vi "5G_PHY_PUSCH_main.vi"() -> ()   [LabVIEW 2015]
uses:
  <vilib>/Utility/miscctls.llb/LVBoundsTypeDef.ctl
  <vilib>/measure/maspectr.llb/FFT Spectrum (Mag-Phase) for 1 Chan (CDB).vi
  <vilib>/measure/NI_MAPro.lvlib
panel:
  out "总比特数 （信宿比特）":dbl
  out "误码率（信源比特和信宿比特比较）":dbl
  out "总比特数（解调制映射输出数据）":dbl
  out "误码率（调制映射输入数据和解调制映射输出数据比较）":dbl
  in  "第1径和第2径相偏(rad)":dbl[](array[numeric])=[0.0, 1.0] min=0.0 max=3.14
  in  "第1径和第2径幅度":dbl[](array[numeric])=[1.0, 0.5] min=0.0 max=1.0
  in  "第1径和第2径频偏(Hz)":dbl[](array[numeric])=[20.0, 140.0] min=0.0 max=180.0
  in  "第1径和第2径时间延迟采样点":dbl[](array[numeric])=[10.0, 140.0] min=0.0 max=200.0
  in  "多径使能":u16(ring) items=["不使能", "使能"]
  out "CRC校验结果":bool
  out "导频2信道估计值":dbl[][](graph)
  out "导频1信道估计值":dbl[][](graph)
  out "OFDM调制后数据（I路）":dbl[](graph)
  out "资源映射后数据（I路）":dbl[][](graph)
  out "产生导频后数据（I路）":dbl[][](graph)
  in  "CP多径时延采样点":i32=140 caption="dB" min=50 max=150
  in  "CP多径时延开关":u16(ring) items=["关", "开"]
  out "接收图片":picture
  out "发送图片":picture
  out "发送信号波形（I路）":dbl[](graph)
  in  "是否添加噪声":u16(ring) items=["关", "开"]
  in  "同步开关":u16(ring)=1 items=["关", "开"]
  in  "频偏(Hz)":i32=120 caption="dB" min=50 max=200
  in  "频偏开关":u16(ring) items=["关", "开"]
  out "相关峰(同步开关打开时显示)":dbl[](graph)
  in  "选择接收图片地址":path=path "C:/Users/DELL/Desktop/5Gphysicallayerlink/01 TeacherVersion/MatlabCode/rx_img.bmp"
  in  "选择发送图片地址":path=path "C:/Users/DELL/Desktop/5Gphysicallayerlink/01 TeacherVersion/MatlabCode/tx_img.bmp"
  out "误码数（调制映射输入数据和解调制映射输出数据比较）":i32
  out "误码数（信源比特和信宿比特比较）":i32
  in  "收发延迟采样点":i32=1400 caption="dB" min=0 max=7000
  in  "收发时延开关":u16(ring) items=["关", "开"]
  in  "突发干扰时域长度":i32=800 caption="dB" min=500 max=1000
  in  "突发干扰开关":u16(ring) items=["关", "开"]
  in  "信道估计开关":u16(ring)=1 items=["关", "开"]
  in  "CP开关":u16(ring)=1 items=["关", "开"]
  in  "交织开关":u16(ring)=1 items=["关", "开"]
  in  "LDPC开关":dbl(ring)=1.0 items=["关", "开"]
  in  "SNR":dbl=17.0 caption="dB" min=-10.0 max=50.0
  out "接收信号波形（I路）":dbl[](graph)
  in  "XSRP IP":string="192.168.1.166"
  in  "PC IP":string="192.168.1.180"
  in  "运行方式":enum16{"仿真运行", "真实系统"}(ring)
  in  "发送参数":T1={"发送通道"=enum."TxCh1", "发送频率"=2380000000.0, "发射衰减 "=40} {"发送频率" format="%#_6p"}
  in  "接收参数":T2={"接收通道"=enum."RxCh1", "接收频率"=2380000000.0, "接收增益 "=20} {"接收频率" format="%#_6p"}
  in  "调制参数":T3={"Nl"=1.0, "subframe_type"=1.0, "cp_type"=0.0, "cfi"=1.0, "UL_subframe_num"=2.0, "prb_num"=100.0, "调制类型"=3, "mimo_type"=1.0} {"调制类型" items=["QPSK"=1, "16QAM"=2, "64QAM"=3, "256QAM"=4]}
  in  "添加噪声":i16(ring) items=["添加噪声"=1, "不添加噪声"=0]
  out "crc_flag":dbl
  out "发送端星座图":cdb[](graph)
  out "接收信号频谱":cluster{"f0":dbl, "df":dbl, "magnitude":dbl[]}(graph)
  out "接收端星座图":cdb[](graph)
  # "基于XSRP软件无线电平台的LTE无线通信系统"
  # "基于XSRP软件无线电平台的5G NR 无线通信系统设计"
  # "实验参数设置"
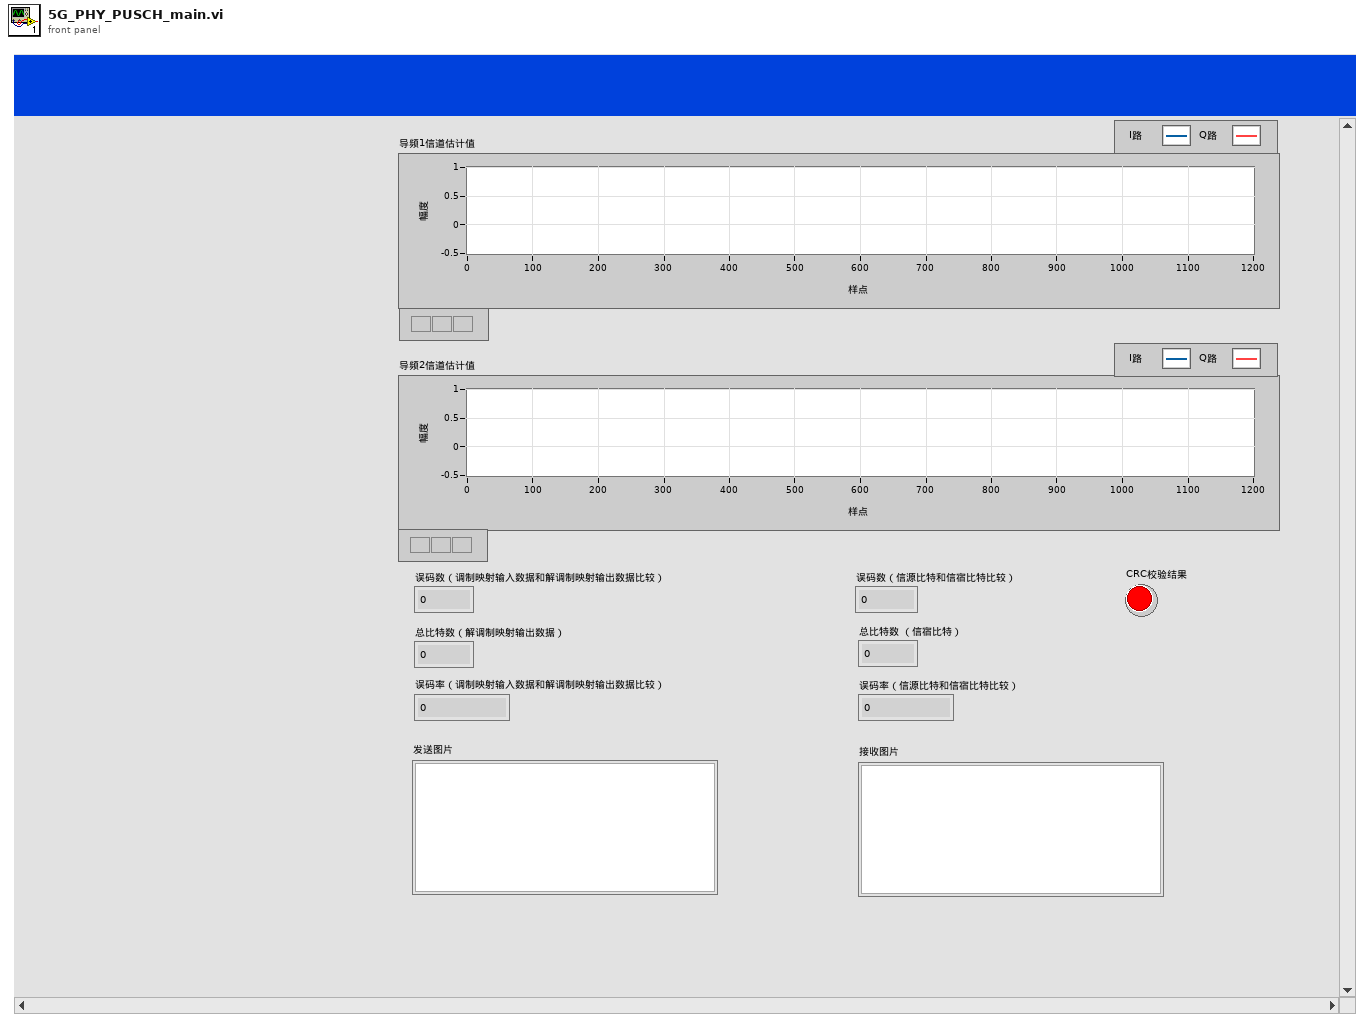
[diagram p1: front panel]
types:
  T1 = cluster{"发送通道":enum16{"TxCh1", "TxCh2"}, "发送频率":dbl, "发射衰减 ":u8}
  T2 = cluster{"接收通道":enum16{"RxCh1", "RxCh2"}, "接收频率":dbl, "接收增益 ":u8}
  T3 = cluster{"Nl":dbl, "subframe_type":dbl, "cp_type":dbl, "cfi":dbl, "UL_subframe_num":dbl, "prb_num":dbl, "调制类型":u16, "mimo_type":dbl}
  T4 = typedef "LVBoundsTypeDef.ctl" = cluster{"Width":u32, "Height":u32}
  T5 = cluster{"dB On (F)":bool, "unwrap phase (F)":bool, "convert to degree (F)":bool}
  T6 = enum8{"Enabled", "Disabled", "Disabled and Grayed Out"}
  T7 = typedef "imagedata.ctl" = cluster{"image type":i32, "image depth":i32, "image":u8[], "mask":u8[], "colors":u32[], "Rectangle":cluster{"left":i16, "top":i16, "right":i16, "bottom":i16}}
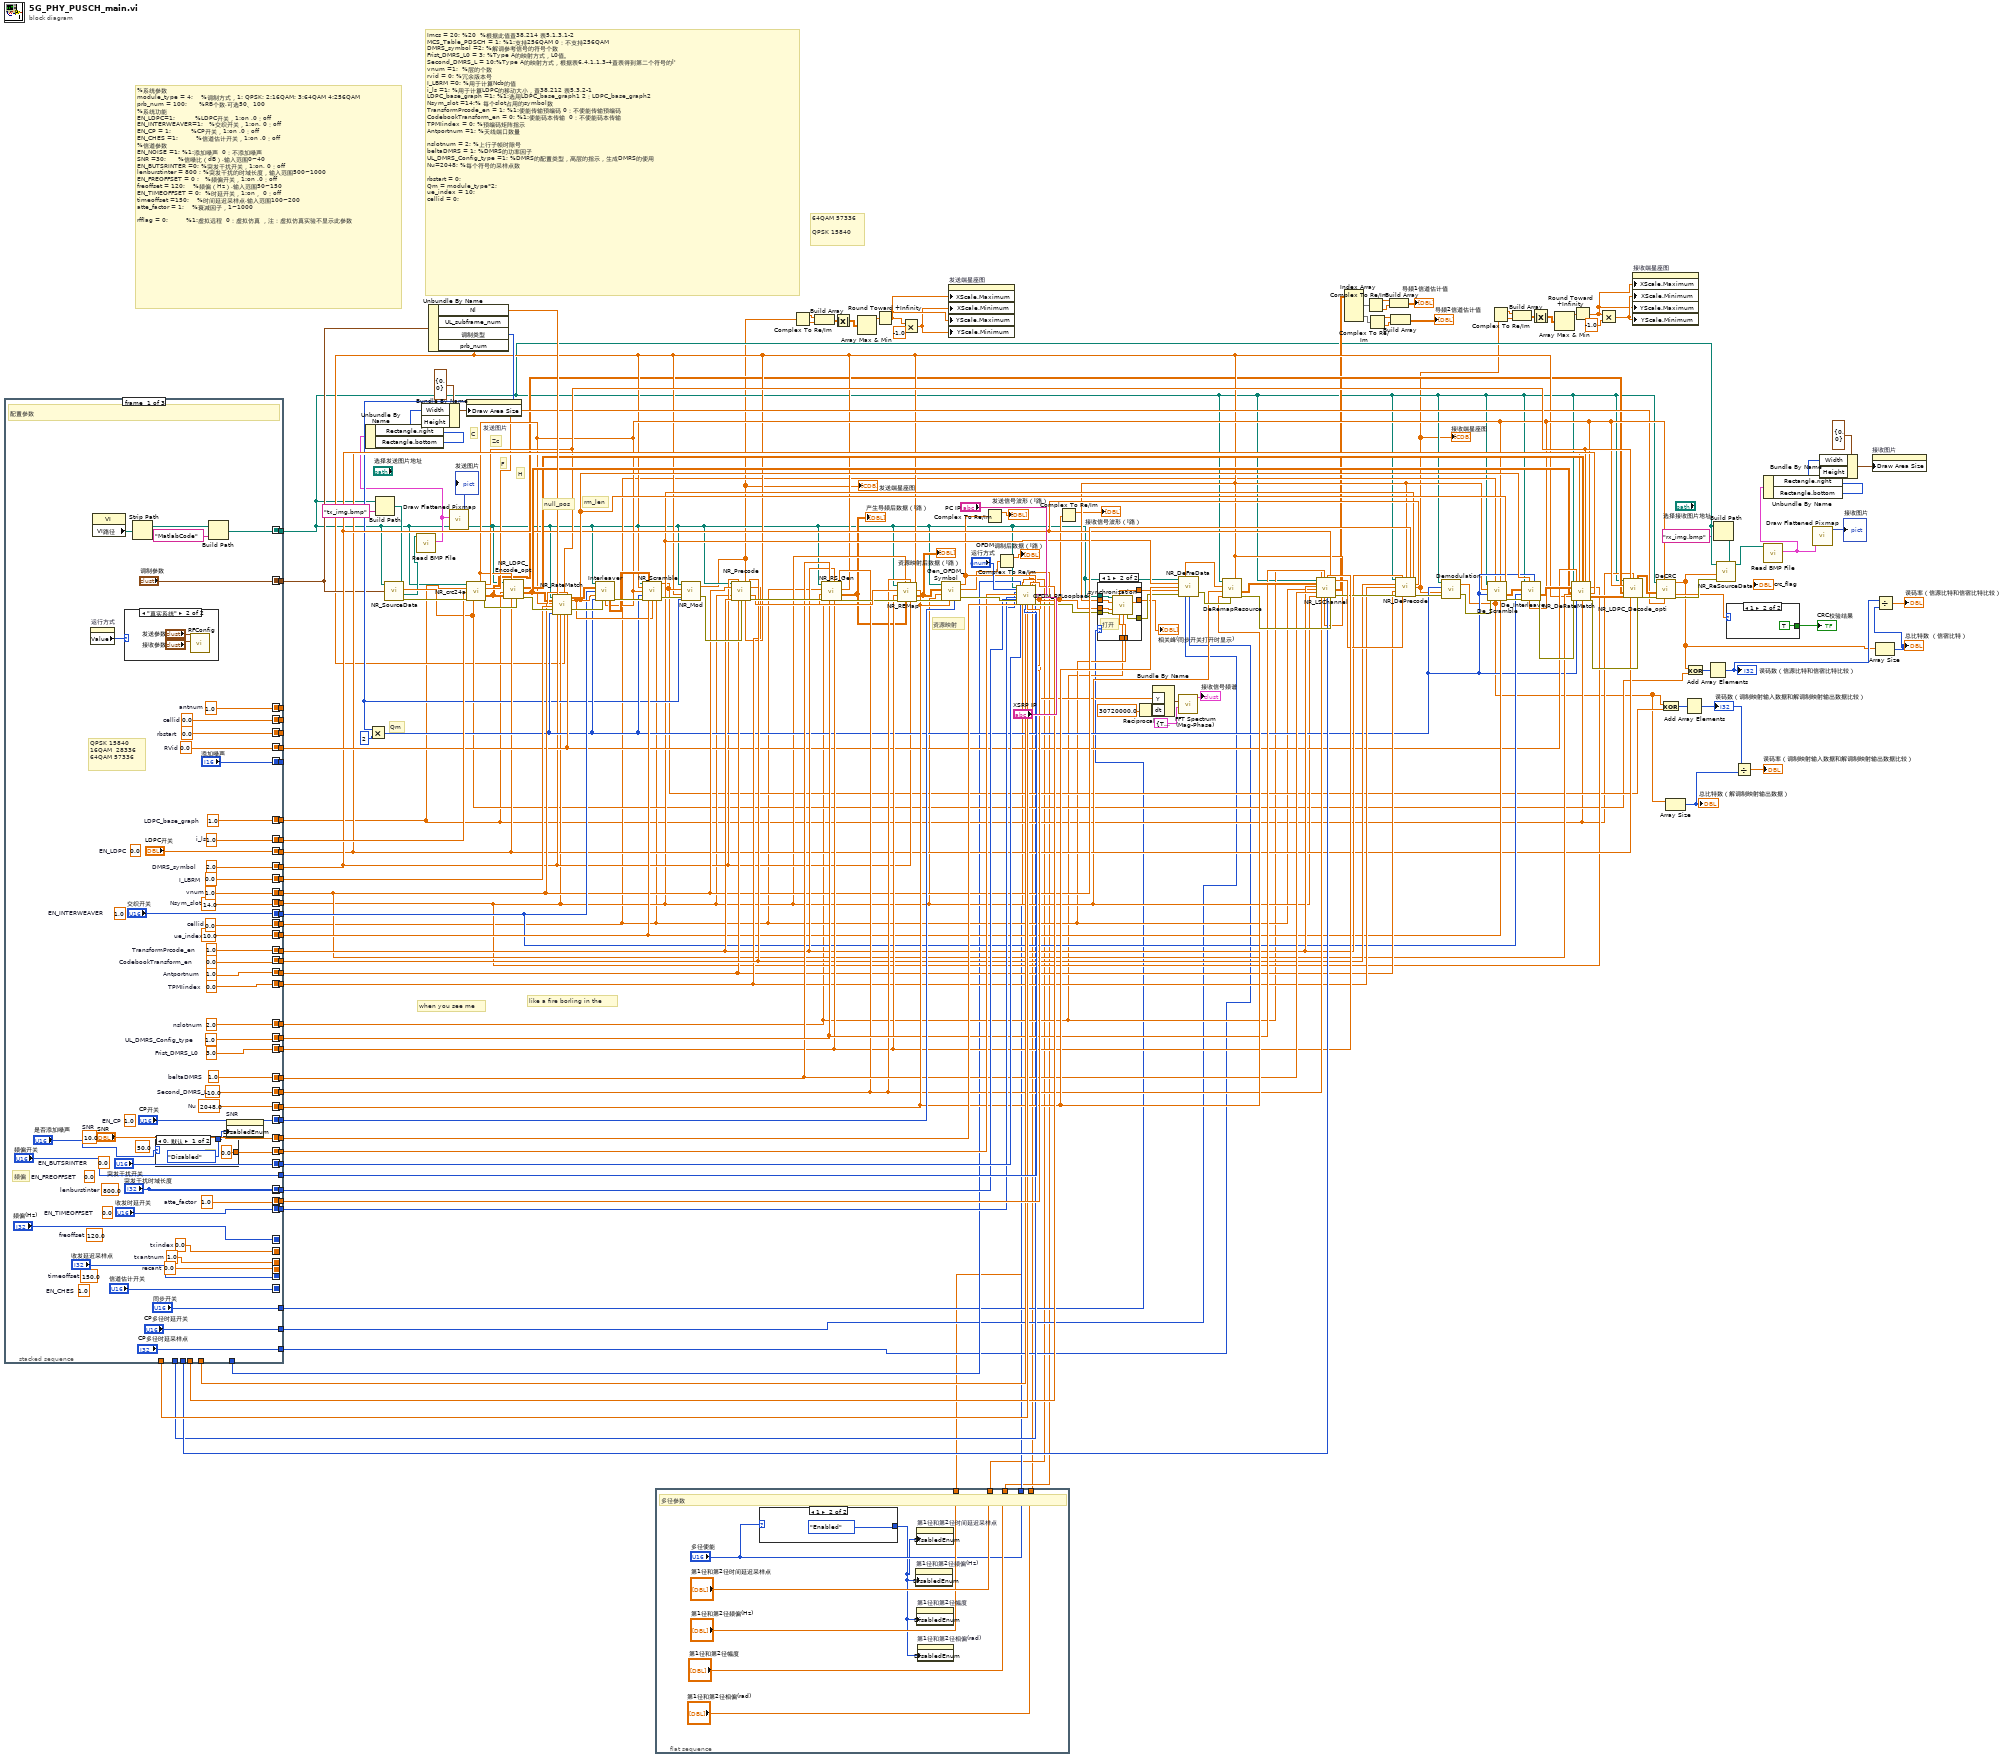
[diagram p0: block diagram]
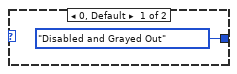
[diagram p2: hidden frame]
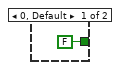
[diagram p3: hidden frame]
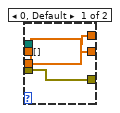
[diagram p4: hidden frame]
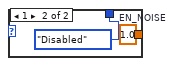
[diagram p5: hidden frame]
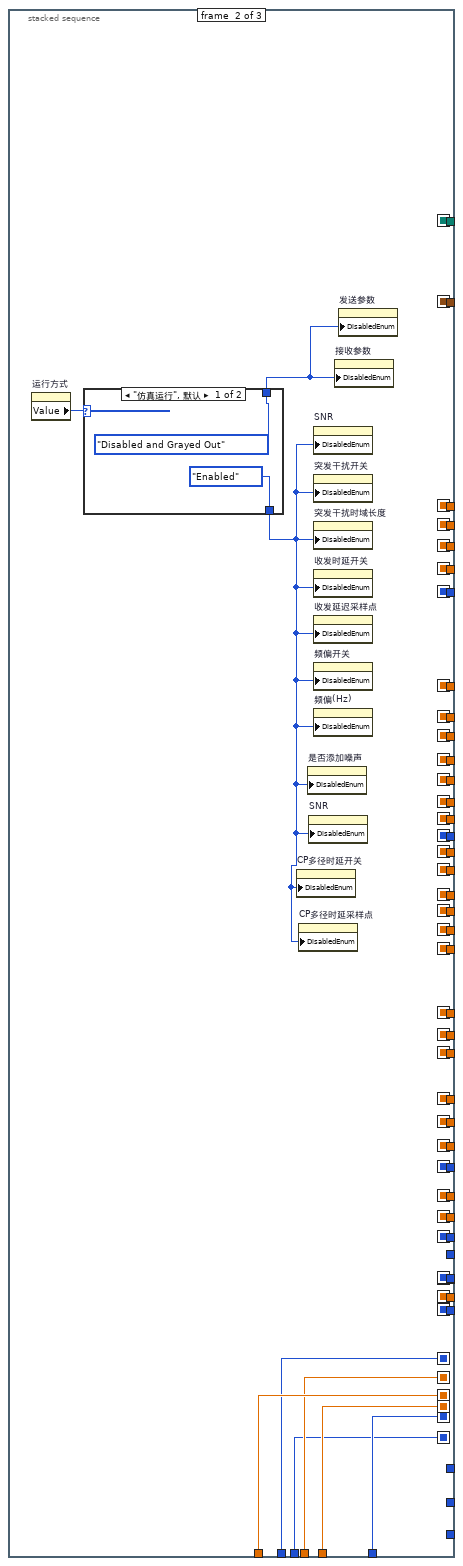
[diagram p7: hidden frame]
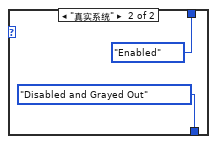
[diagram p8: hidden frame]
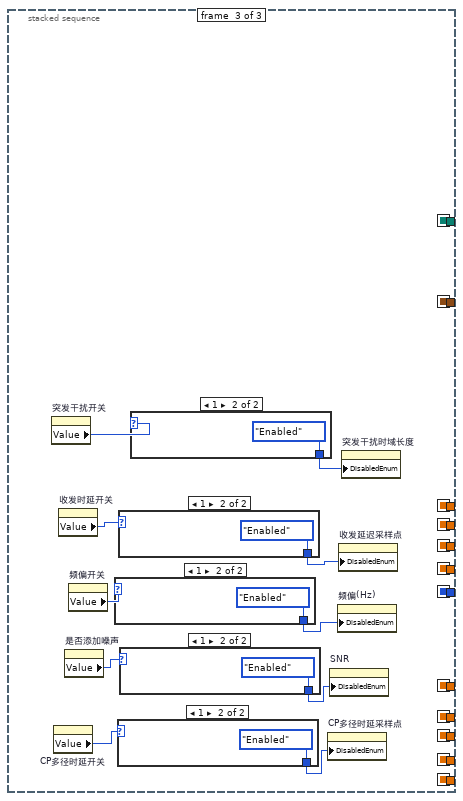
[diagram p9: hidden frame]
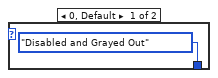
[diagram p10: hidden frame]
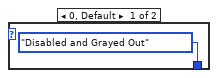
[diagram p11: hidden frame]
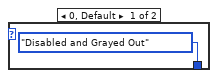
[diagram p12: hidden frame]
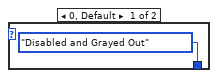
[diagram p13: hidden frame]
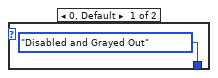
[diagram p14: hidden frame]
diagram:
  # "like a fire borling in the"
  # "when you see me"
  # "rm_len"
  # "Qm"
  # "null_pos"
  # "H"
  # "F"
  # "Zc"
  # "C"
  # "%系统参数\nmodule_type = 4;    %调制方式，1: QPSK; 2:16QAM; 3:64QAM 4:256QAM\nprb_num = 100;      %RB个数,可选50、100\n%系统功能\nEN_LDPC=1;          %LDPC开关，1:on ,0：off\nEN_INTERWEAVER=1;   %交织开关，1:on, 0：off\nEN_CP = 1;          %CP开关，1:on ,0：off\nEN_CHES =1;         %信道估计开关，1:on ,0：off \n%信道参数\nEN_NOISE =1; %1:添加噪声  0：不添加噪声\nSNR =30;      %信噪比（dB）,输入范围0~40\nEN_BUTSRINTER =0; %突发干扰开关，1:on, 0：off\nlenburstinter = 800 ; %突发干扰的时域长度，输入范围500~1000\nEN_FREOFFSET = 0 ;   %频偏开关，1:on ,0：off\nfreoffset = 120;    %频偏（Hz）,输入范围50~150\nEN_TIMEOFFSET = 0;  %时延开关，1:on， 0：off\ntimeoffset =150;    %时间延迟采样点,输入范围100~200\natte_factor = 1;    %衰减因子，1~1000\n\nrfflag = 0;         %1:虚拟远程  0：虚拟仿真 ，注：虚拟仿真实验不显示此参数"
  # "Imcs = 20; %20  %根据此值查38.214 表5.1.3.1-2\nMCS_Table_PDSCH = 1; %1:支持256QAM 0：不支持256QAM\nDMRS_symbol =2; %解调参考信号的符号个数\nFrist_DMRS_L0 = 3; %Type A的映射方式，L0值。\nSecond_DMRS_L = 10;%Type A的映射方式，根据表6.4.1.1.3-4查表得到第二个符号的l'\nvnum =1;  %层的个数\nrvid = 0; %冗余版本号\nI_LBRM =0; %用于计算Ncb的值\ni_ls =1; %用于计算LDPC的移动大小，查38.212 表5.3.2-1\nLDPC_base_graph =1; %1:选用LDPC_base_graph1 2：LDPC_base_graph2\nNsym_slot =14;% 每个slot占用的symbol数\nTransformPrcode_en = 1; %1:使能传输预编码 0：不使能传输预编码\nCodebookTransform_en = 0; %1:使能码本传输  0：不使能码本传输\nTPMIindex = 0; %预编码矩阵指示\nAntportnum =1; %天线端口数量\n\nnslotnum = 2; %上行子帧时隙号\nbeltaDMRS = 1; %DMRS的功率因子\nUL_DMRS_Config_type =1; %DMRS的配置类型，高层的指示，生成DMRS的使用\nNu=2048; %每个符号的采样点数\n\nrbstart = 0;\nQm = module_type*2;\nue_index = 10;\ncellid = 0;"
  # "资源映射"
  # "64QAM 57336\n\nQPSK 15840"
  n1 = stacked-sequence {
    seq-local: ["调制参数" _ _] -> [_ w267 _]
    seq-local: [w209 _ _] -> [_ w266 _]
    seq-local: [w214 _ _] -> [_ w265 _]
    seq-local: [w211 _ _] -> [_ w264 _]
    seq-local: [w215 _ _] -> [_ w263 _]
    seq-local: [w216 _ _] -> [_ w262 _]
    seq-local: [w213 _ _] -> [_ w261 _]
    seq-local: [w210 _ _] -> [_ w260 _]
    seq-local: ["添加噪声" _ _] -> [_ w259 _]
    seq-local: [w212 _ _] -> [_ w258 _]
    seq-local: [w205 _ _] -> [_ w257 _]
    seq-local: [w203 _ _] -> [_ w256 _]
    seq-local: [w202 _ _] -> [_ w255 _]
    seq-local: ["LDPC开关" _ _] -> [_ w254 _]
    seq-local: [w201 _ _] -> [_ w253 _]
    seq-local: ["交织开关" _ _] -> [_ w252 _]
    seq-local: [w200 _ _] -> [_ w251 _]
    seq-local: [w199 _ _] -> [_ w250 _]
    seq-local: [w198 _ _] -> [_ w249 _]
    seq-local: [w197 _ _] -> [_ w248 _]
    seq-local: [w196 _ _] -> [_ w247 _]
    seq-local: [w195 _ _] -> [_ w246 _]
    seq-local: [w194 _ _] -> [_ w245 _]
    seq-local: [w193 _ _] -> [_ w244 _]
    seq-local: [w192 _ _] -> [_ w243 _]
    seq-local: [w191 _ _] -> [_ w242 _]
    seq-local: [w190 _ _] -> [_ w241 _]
    seq-local: ["SNR" _ _] -> [_ w240 _]
    seq-local: [w189 _ _] -> [_ w239 _]
    seq-local: ["突发干扰开关" _ _] -> [_ w238 _]
    seq-local: ["突发干扰时域长度" _ _] -> [_ w237 _]
    seq-local: ["突发干扰时域长度" _ _] -> [_ w236 _]
    seq-local: [w188 _ _] -> [_ w235 _]
    seq-local: ["收发时延开关" _ _] -> [_ w234 _]
    seq-local: ["收发延迟采样点" _ _] -> [_ w233 _]
    seq-local: [w186 _ _] -> [_ w232 _]
    seq-local: [w187 _ _] -> [_ w231 _]
    seq-local: [w185 _ _] -> [_ w230 _]
    seq-local: ["CP开关" _ _] -> [_ w229 _]
    seq-local: ["频偏(Hz)" _ _] -> [_ w228 _]
    seq-local: ["信道估计开关" _ _] -> [_ w227 _]
    tunnel: [_ w267 _] -> w89
    tunnel: [_ w266 _] -> _
    tunnel: [_ w265 _] -> w163
    tunnel: [_ w264 _] -> w102
    tunnel: [_ w263 _] -> w103
    tunnel: [_ w262 _] -> w97
    tunnel: [_ w261 _] -> w109
    tunnel: [_ w260 _] -> _
    tunnel: [_ w259 _] -> _
    tunnel: [_ w258 _] -> _
    tunnel: [_ w257 _] -> w39
    tunnel: [_ w256 _] -> w74
    tunnel: [_ w255 _] -> w145
    tunnel: [_ w254 _] -> w95
    tunnel: [_ w253 _] -> w90
    tunnel: [_ w252 _] -> w105
    tunnel: [_ w251 _] -> w78
    tunnel: [_ w250 _] -> w111
    tunnel: [_ w249 _] -> w114
    tunnel: [_ w248 _] -> w112
    tunnel: [_ w247 _] -> w113
    tunnel: [_ w246 _] -> w77
    tunnel: [_ w245 _] -> w121
    tunnel: [_ w244 _] -> w117
    tunnel: [_ w243 _] -> w120
    tunnel: [_ w242 _] -> w119
    tunnel: [_ w241 _] -> w124
    tunnel: [_ w240 _] -> w136
    tunnel: [_ w239 _] -> w135
    tunnel: [_ w238 _] -> w134
    tunnel: ["频偏开关" _ _] -> w133
    tunnel: [_ w237 _] -> _
    tunnel: [_ w236 _] -> w132
    tunnel: [_ w235 _] -> w131
    tunnel: [_ w234 _] -> w130
    tunnel: [_ w233 _] -> w72
    tunnel: [_ w232 _] -> w129
    tunnel: [_ w231 _] -> w128
    tunnel: [_ w230 _] -> w127
    tunnel: [_ w229 _] -> w126
    tunnel: [_ w228 _] -> w73
    tunnel: [_ w227 _] -> w118
    tunnel: ["同步开关" _ _] -> w71
    tunnel: ["CP多径时延开关" _ _] -> w66
    tunnel: ["CP多径时延采样点" _ _] -> w65
    frame #0 {
      (unwired) 50.0 ("y")
      (unwired) 1.0  # EN_CHES
      (unwired) 120.0  # freoffset
      (unwired) 1.0  # EN_CP
      w185 = 0.0  # txindex
      w186 = 1.0  # txantnum
      w187 = 0.0  # recant
      (unwired) 150.0  # timeoffset
      (unwired) 0.0  # EN_TIMEOFFSET
      w188 = 1.0  # atte_factor
      (unwired) 800.0  # lenburstinter
      (unwired) 0.0  # EN_FREOFFSET
      (unwired) 0.0  # EN_BUTSRINTER
      (unwired) 10.0  # SNR
      w190 = 2048.0  # Nu
      w191 = 10.0  # Second_DMRS_L
      w192 = 1.0  # beltaDMRS
      w193 = 3.0  # Frist_DMRS_L0
      w194 = 1.0  # UL_DMRS_Config_type
      w195 = 2.0  # nslotnum
      w196 = 0.0  # TPMIindex
      w197 = 1.0  # Antportnum
      w198 = 0.0  # CodebookTransform_en
      w199 = 1.0  # TransformPrcode_en
      w200 = 0.0  # cellid
      (unwired) 1.0  # EN_INTERWEAVER
      w201 = 14.0  # Nsym_slot
      (unwired) 0.0  # EN_LDPC
      w202 = 1.0  # i_ls
      w203 = 1.0  # LDPC_base_graph
      w209 = 0.0  # cellid
      w210 = 0.0  # rbstart
      w211 = 0.0  # RVid
      w212 = 1.0  # antnum
      w213 = 10.0  # ue_index
      w214 = 0.0  # I_LBRM
      w215 = 1.0  # vnum
      w216 = 2.0  # DMRS_symbol
      # "频偏"
      # "QPSK 15840\n16QAM  28336\n64QAM 57336"
      # "配置参数"
      n2 = property on="运行方式" class="Enum (严格)"() -> ("Value"=w184:enum16{"仿真运行", "真实系统"})  [unwired: 2 in, 2 out]
      n3 = property class="VI"() -> ("VI路径"=w206:path)  [unwired: 2 in, 2 out]
      n4 = case shown="\"真实系统\"" w184 {
        frame "仿真运行", Default {
        }
        frame "真实系统" {
          n5 = call "RFConfig.vi"("接收参数设置"="接收参数", "发射参数设置"="发送参数") -> ()  [unwired: 9 in, 1 out]
        }
      }
      n6 = Strip Path(path=w206) -> (stripped path=w207:path)  [unwired: 1 out]
      n7 = case shown="0, 默认" "是否添加噪声" {
        tunnel: [0.0 ("EN_NOISE") w221] -> w189
        tunnel: [T6."Disabled" ("禁用") T6."Disabled" ("禁用")] -> w168
        frame 0, Default {
          # "关"
        }
        frame 1 {
          w221 = 1.0  # EN_NOISE
        }
      }
      n8 = Build Path(base path=w207, name or relative path="MatlabCode") -> (appended path=w205:path)
      n9 = property on="SNR" class="DigNum (严格)"("DisabledEnum"=w168) -> ()  [unwired: 2 in, 2 out]
    }
    frame #1 {
      n10 = property on="运行方式" class="Enum (严格)"() -> ("Value"=w226:enum16{"仿真运行", "真实系统"})  [unwired: 2 in, 2 out]
      n11 = case shown="\"仿真运行\", 默认" w226 {
        tunnel: [T6."Enabled" ("禁用") T6."Disabled and Grayed Out" ("禁用")] -> w224
        tunnel: [T6."Disabled and Grayed Out" ("禁用") T6."Enabled" ("禁用")] -> w225
        frame "仿真运行", Default {
        }
        frame "真实系统" {
        }
      }
      n12 = property on="CP多径时延开关" class="Ring (严格)"("DisabledEnum"=w224) -> ()  [unwired: 2 in, 2 out]
      n13 = property on="CP多径时延采样点" class="DigNum (严格)"("DisabledEnum"=w224) -> ()  [unwired: 2 in, 2 out]
      n14 = property on="是否添加噪声" class="Ring (严格)"("DisabledEnum"=w224) -> ()  [unwired: 2 in, 2 out]
      n15 = property on="SNR" class="DigNum (严格)"("DisabledEnum"=w224) -> ()  [unwired: 2 in, 2 out]
      n16 = property on="SNR" class="DigNum (严格)"("DisabledEnum"=w224) -> ()  [unwired: 2 in, 2 out]
      n17 = property on="突发干扰开关" class="Ring (严格)"("DisabledEnum"=w224) -> ()  [unwired: 2 in, 2 out]
      n18 = property on="突发干扰时域长度" class="DigNum (严格)"("DisabledEnum"=w224) -> ()  [unwired: 2 in, 2 out]
      n19 = property on="收发时延开关" class="Ring (严格)"("DisabledEnum"=w224) -> ()  [unwired: 2 in, 2 out]
      n20 = property on="收发延迟采样点" class="DigNum (严格)"("DisabledEnum"=w224) -> ()  [unwired: 2 in, 2 out]
      n21 = property on="频偏开关" class="Ring (严格)"("DisabledEnum"=w224) -> ()  [unwired: 2 in, 2 out]
      n22 = property on="频偏(Hz)" class="DigNum (严格)"("DisabledEnum"=w224) -> ()  [unwired: 2 in, 2 out]
      n23 = property on="接收参数" class="Clust (严格)"("DisabledEnum"=w225) -> ()  [unwired: 2 in, 2 out]
      n24 = property on="发送参数" class="Clust (严格)"("DisabledEnum"=w225) -> ()  [unwired: 2 in, 2 out]
    }
    frame #2 {
      n25 = property on="突发干扰开关" class="Ring (严格)"() -> ("Value"=w281:u16)  [unwired: 2 in, 2 out]
      n26 = property on="CP多径时延开关" class="Ring (严格)"() -> ("Value"=w273:u16)  [unwired: 2 in, 2 out]
      n27 = property on="收发时延开关" class="Ring (严格)"() -> ("Value"=w278:u16)  [unwired: 2 in, 2 out]
      n28 = property on="是否添加噪声" class="Ring (严格)"() -> ("Value"=w276:u16)  [unwired: 2 in, 2 out]
      n29 = property on="频偏开关" class="Ring (严格)"() -> ("Value"=w272:u16)  [unwired: 2 in, 2 out]
      n30 = case shown="1" w272 {
        tunnel: [T6."Disabled and Grayed Out" ("禁用") T6."Enabled" ("禁用")] -> w277
        frame 0, Default {
        }
        frame 1 {
        }
      }
      n31 = case shown="1" w273 {
        tunnel: [T6."Disabled and Grayed Out" ("禁用") T6."Enabled" ("禁用")] -> w274
        frame 0, Default {
        }
        frame 1 {
        }
      }
      n32 = case shown="1" w278 {
        tunnel: [T6."Disabled and Grayed Out" ("禁用") T6."Enabled" ("禁用")] -> w279
        frame 0, Default {
        }
        frame 1 {
        }
      }
      n33 = case shown="1" w276 {
        tunnel: [T6."Disabled and Grayed Out" ("禁用") T6."Enabled" ("禁用")] -> w275
        frame 0, Default {
        }
        frame 1 {
        }
      }
      n34 = case shown="1" w281 {
        tunnel: [T6."Disabled and Grayed Out" ("禁用") T6."Enabled" ("禁用")] -> w280
        frame 0, Default {
        }
        frame 1 {
        }
      }
      n35 = property on="CP多径时延采样点" class="DigNum (严格)"("DisabledEnum"=w274) -> ()  [unwired: 2 in, 2 out]
      n36 = property on="SNR" class="DigNum (严格)"("DisabledEnum"=w275) -> ()  [unwired: 2 in, 2 out]
      n37 = property on="频偏(Hz)" class="DigNum (严格)"("DisabledEnum"=w277) -> ()  [unwired: 2 in, 2 out]
      n38 = property on="收发延迟采样点" class="DigNum (严格)"("DisabledEnum"=w279) -> ()  [unwired: 2 in, 2 out]
      n39 = property on="突发干扰时域长度" class="DigNum (严格)"("DisabledEnum"=w280) -> ()  [unwired: 2 in, 2 out]
    }
  }
  n40 = Build Path(base path=w39, name or relative path="tx_img.bmp" ("名称或相对路径")) -> (appended path=w42:path)
  n41 = call "NR_SourceData.vi"("appended path"=w39, "ParametersCluster"=w89, "imagestxpath"=w42) -> ("info_data"=w85:dbl[], "imagessendpath"=w43:path, "error IO"=w152:errorcluster)  [unwired: 1 in]
  n42 = call <vilib>:"Read BMP File.vi"("path to BMP file"=w43) -> ("image data"=w53:T7)  [unwired: 8 in, 2 out]
  n43 = Unbundle By Name(w53) -> ("Rectangle.right"=w52:i16, "Rectangle.bottom"=w51:i16)
  n44 = Bundle By Name(cluster=T4 {"Width"=0, "Height"=0} ("绘图区域大小"), "Width"=w52, "Height"=w51) -> (w50:T4)
  n45 = Unbundle By Name(w89) -> ("Nl"=w164:dbl, "调制类型"=w91:u16, "prb_num"=w80:dbl)  [unwired: 1 out]
  n46 = Multiply(x=w91, y=u16 2) -> (x*y=w101:u16)
  n47 = call <vilib>:"Draw Flattened Pixmap.vi"("image data"=w53) -> ("new picture"=→"发送图片":picture)  [unwired: 8 in]
  n48 = call "NR_crc24a.vi"("appended path"=w39, "LDPC_base_graph"=w74, "i_ls"=w145, "error in (no error)"=w152, "info_data"=w85) -> ("C"=w93:dbl, "Zc"=w96:dbl, "F"=w92:dbl, "cdblkseg_data"=w75:dbl[][], "error out"=w144:errorcluster)  [unwired: 6 in]
  n49 = property on="发送图片" class="Pict"("Draw Area Size"=w50) -> ()  [unwired: 2 in, 2 out]
  n50 = call "NR_LDPC_Encode_opt.vi"("error in (no error)"=w144, "EN_LDPC"=w95, "C"=w93, "cdblkseg_data"=w75, "LDPC_base_graph"=w74, "appended path"=w39) -> ("error out"=w167:errorcluster, "coded_data"=w100:dbl[][], "null_pos"=w99:dbl[][])  [unwired: 2 in, 1 out]
  n51 = call "NR_RateMatch.vi"("PA"=w39, "coded_data"=w100, "C"=w93, "I_LBRM"=w163, "error in (no error)"=w167, "Qm"=w101, "LDPC_base_graph"=w164, "DMRS_symbol"=w97, "Nsym_slot"=w90, "Zc"=w96, "prb_num"=w80, "vnum"=w103, "rvid"=w102) -> ("rm_data"=w106:dbl[][], "rm_len"=w107:dbl[], "error out"=w142:errorcluster)  [unwired: 4 in]
  n52 = call "Interleaver.vi"("appended path"=w39, "rm_data"=w106, "EN_INTERWEAVER"=w105, "rm_len"=w107, "Qm"=w101, "error in (no error)"=w142, "C"=w93) -> ("error out"=w166:errorcluster, "iw_data"=w141:dbl[][])  [unwired: 7 in]
  n53 = call "NR_Scramble.vi"("appended path"=w39, "iw_data"=w141, "prb_num"=w80, "C"=w93, "Qm"=w101, "error in (no error)"=w166, "ue_index"=w109, "rm_len"=w107, "cellid"=w78) -> ("scramble_data"=w88:dbl[], "error out"=w165:errorcluster)  [unwired: 5 in]
  n54 = flat-sequence {
    tunnel: ["多径使能"] -> w13
    tunnel: ["第1径和第2径时间延迟采样点"] -> w12
    tunnel: ["第1径和第2径频偏(Hz)"] -> w11
    tunnel: ["第1径和第2径幅度"] -> w10
    tunnel: ["第1径和第2径相偏(rad)"] -> w9
    frame #0 {
      # "多径参数"
      n55 = case shown="1" "多径使能" {
        tunnel: [T6."Disabled and Grayed Out" ("Disabled") T6."Enabled" ("Disabled")] -> w292
        frame 0, Default {
        }
        frame 1 {
        }
      }
      n56 = property on="第1径和第2径频偏(Hz)" class="Arr (严格)"("DisabledEnum"=w292) -> ()  [unwired: 2 in, 2 out]
      n57 = property on="第1径和第2径时间延迟采样点" class="Arr (严格)"("DisabledEnum"=w292) -> ()  [unwired: 2 in, 2 out]
      n58 = property on="第1径和第2径幅度" class="Arr (严格)"("DisabledEnum"=w292) -> ()  [unwired: 2 in, 2 out]
      n59 = property on="第1径和第2径相偏(rad)" class="Arr (严格)"("DisabledEnum"=w292) -> ()  [unwired: 2 in, 2 out]
    }
  }
  n60 = call "NR_Mod.vi"("appended path"=w39, "scramble_data"=w88, "prb_num"=w80, "module_type"=w91, "error in (no error)"=w165) -> ("mod_data"=w37:cdb[], "error out"=w150:errorcluster)
  "发送端星座图" <- w37
  n61 = call "NR_Precode.vi"("appended path"=w39, "DMRS_symbol"=w97, "mod_data"=w37, "CodebookTransform_en"=w114, "vnum"=w103, "TPMIindex"=w113, "Nsym_slot"=w90, "TransformPrcode_en"=w111, "Antportnum"=w112, "error in (no error)"=w150, "prb_num"=w80) -> ("precodedata"=w140:cdb[], "error IO"=w151:errorcluster)  [unwired: 3 in]
  n62 = Complex To Re/Im(x + iy=w37) -> (x=w36:dbl[], y=w35:dbl[])
  n63 = Build Array(w36, w35) -> (w34:dbl[][])
  n64 = call "NR_RS_Gen.vi"("prb_num"=w80, "Second_DMRS_L"=w119, "Frist_DMRS_L0"=w117, "TransformPrcode_en"=w111, "UL_DMRS_Config_type"=w121, "beltaDMRS"=w120, "error in (no error)"=w151, "nslotnum"=w77, "cellid"=w78, "appended path"=w39) -> ("error IO"=w139:errorcluster, "rsdata"=w64:cdb[][])
  "产生导频后数据（I路）" <- w64
  n65 = Absolute Value(x=w34) -> (abs(x)=w33:dbl[][])
  n66 = Array Max & Min(array=w33) -> (max value=w32:dbl)  [unwired: 3 out]
  n67 = Round Toward +Infinity(x=w32) -> (ceil(x): smallest int >= x=w31:dbl)
  n68 = call "NR_REMap.vi"("Nu"=w124, "prb_num"=w80, "DMRS_symbol"=w97, "Second_DMRS_L"=w119, "rsdata"=w64, "Nsym_slot"=w90, "error in (no error)"=w139, "Frist_DMRS_L0"=w117, "precodedata"=w140, "appended path"=w39) -> ("error IO"=w138:errorcluster, "fredata"=w63:cdb[][])
  "资源映射后数据（I路）" <- w63
  n69 = Multiply(x=w31, y=-1.0) -> (x*y=w30:dbl)
  n70 = call "Gen_OFDM_Symbol.vi"("EN_CP"=w126, "Nu"=w124, "error in (no error)"=w138, "Nsym_slot"=w90, "fredata"=w63, "appended path"=w39) -> ("error IO"=w158:errorcluster, "input"=w16:cdb[], "txdata"=w70:cdb[])  [unwired: 1 in]
  n71 = property on="发送端星座图" class="XYGraph (严格)"("XScale.Maximum"=w31, "XScale.Minimum"=w30, "YScale.Maximum"=w31, "YScale.Minimum"=w30) -> ()  [unwired: 2 in, 2 out]
  n72 = Complex To Re/Im(x + iy=w70) -> (x=→"发送信号波形（I路）":dbl[])  [unwired: 1 out]
  n73 = Complex To Re/Im(x + iy=w16) -> (x=→"OFDM调制后数据（I路）":dbl[])  [unwired: 1 out]
  n74 = call "OFDM_RFLoopback.vi"("PathIn"=w39, "rfflag"="运行方式", "EN_Mutipath"=w13, "EN_NOISE"=w135, "EN_TIMEOFFSET"=w130, "lenburstinter"=w132, "SNR"=w136, "timeoffset"=w72, "EN_BUTSRINTER"=w134, "mutitimeoffset"=w12, "mutifreoffset"=w11, "recant"=w128, "EN_FREOFFSET"=w133, "txantnum"=w129, "atte_factor"=w131, "txindex"=w127, "error in (no error)"=w158, "mutiamp"=w10, "mutiphaseoffset"=w9, "txdata"=w70, "freoffset"=w73, "pcip"="PC IP", "xsrpip"="XSRP IP") -> ("rxdata"=w79:cdb[], "error out"=w83:errorcluster)  [unwired: 3 in]
  n75 = Complex To Re/Im(x + iy=w79) -> (x=→"接收信号波形（I路）":dbl[])  [unwired: 1 out]
  n76 = case shown="1" w71 {
    tunnel: w83 -> [w301 w311]
    tunnel: [w301 w310] -> w82
    tunnel: [w302 w309] -> w81
    tunnel: w39 -> [_ w308]
    tunnel: w80 -> [_ w307]
    tunnel: w79 -> [w302 w306]
    tunnel: w78 -> [_ w305]
    tunnel: w77 -> [_ w304]
    tunnel: [dbl[] [] ("corrdata") w303] -> w76
    frame 0, Default {
    }
    frame 1 {
      # "打开"
      n77 = call "synchronization .vi"("appended path"=w308, "prb_num"=w307, "rxData"=w306, "error in (no error)"=w311, "UL_subframe_num"=w304, "cellid"=w305) -> ("rxmodify"=w309:cdb[], "corrdata"=w303:dbl[], "error IO"=w310:errorcluster)  [unwired: 6 in, 1 out]
    }
  }
  "相关峰(同步开关打开时显示)" <- w76
  n78 = Reciprocal(x=30720000.0) -> (1/x=w155:dbl)
  n79 = Bundle By Name("Y"=w79, "dt"=w155) -> (w157:waveform(cdb))  [unwired: 1 in]
  n80 = call-poly <vilib>:"FFT Spectrum (Mag-Phase).vi"("view"=T5 {"dB On (F)"=TRUE, "unwrap phase (F)"=FALSE, "convert to degree (F)"=FALSE}, "time signal"=w157) -> ("magnitude"=→"接收信号频谱":cluster{"f0":dbl, "df":dbl, "magnitude":dbl[]})  [unwired: 5 in, 4 out]
  n81 = call "NR_DeFreData .vi"("appended path"=w39, "Nsym_slot,"=w90, "Nu"=w124, "rxdata"=w81, "error in (no error)"=w82, "EN_TIMEOFFSETCP"=w66, "timeoffsetCP"=w65) -> ("defredata"=w125:cdb[], "error IO"=w147:errorcluster)  [unwired: 7 in]
  n82 = call "DeRemapResource.vi"("prb_num"=w80, "error in (no error)"=w147, "Nu"=w124, "Nsym_slot"=w90, "defredata"=w125, "appended path"=w39) -> ("error IO"=w122:errorcluster, "deremapdata"=w123:cdb[][])  [unwired: 3 in]
  n83 = call "NR_LSChannel.vi"("appended path"=w39, "deremapdata"=w123, "TransformPrcode_en"=w111, "cellid"=w78, "beltaDMRS"=w120, "Nsym_slot"=w90, "nslotnum"=w77, "Second_DMRS_L"=w119, "UL_DMRS_Config_type"=w121, "prb_num"=w80, "Frist_DMRS_L0"=w117, "EN_CHES"=w118, "DMRS_symbol"=w97, "error in (no error)"=w122) -> ("equdata"=w116:cdb[], "slotlschanneldata"=w62:cdb[][], "error IO"=w115:errorcluster)  [unwired: 3 in]
  n84 = Index Array(array=w62) -> (element #1=w61:cdb[], element #2=w54:cdb[])  [unwired: 4 in]
  n85 = Complex To Re/Im(x + iy=w61) -> (x=w60:dbl[], y=w57:dbl[])
  n86 = Complex To Re/Im(x + iy=w54) -> (x=w56:dbl[], y=w58:dbl[])
  n87 = Build Array(w60, w57) -> (→"导频1信道估计值":dbl[][])
  n88 = Build Array(w56, w58) -> (→"导频2信道估计值":dbl[][])
  n89 = call "NR_DePrecode.vi"("appended path"=w39, "TransformPrcode_en"=w111, "prb_num"=w80, "vnum"=w103, "Nsym_slot"=w90, "CodebookTransform_en"=w114, "DMRS_symbol"=w97, "TPMIindex"=w113, "Antportnum"=w112, "error in (no error)"=w115, "equdata"=w116) -> ("delayermapdata"=w22:cdb[], "error IO"=w110:errorcluster)  [unwired: 3 in]
  "接收端星座图" <- w22
  n90 = call "Demodulation.vi"("error in (no error)"=w110, "delayermapdata"=w22, "Qm"=w101, "appended path"=w39) -> ("error IO"=w162:errorcluster, "demoddata"=w3:dbl[])
  n91 = call "De_Scramble.vi"("rm_len"=w107, "ue_index"=w109, "C"=w93, "demoddata"=w3, "cellid"=w78, "error in (no error)"=w162, "Qm"=w101, "prb_num"=w80, "appended path"=w39) -> ("error IO"=w161:errorcluster, "deccbc_data"=w108:dbl[][])  [unwired: 1 in]
  n92 = Complex To Re/Im(x + iy=w22) -> (x=w23:dbl[], y=w24:dbl[])
  n93 = Build Array(w23, w24) -> (w25:dbl[][])
  n94 = call "De_Interleave.vi"("Qm"=w101, "C"=w93, "rm_len"=w107, "error in (no error)"=w161, "EN_INTERWEAVER"=w105, "deccbc_data"=w108, "appended path"=w39) -> ("error IO"=w160:errorcluster, "deiwdata"=w104:dbl[][])  [unwired: 3 in]
  n95 = Absolute Value(x=w25) -> (abs(x)=w26:dbl[][])
  n96 = Array Max & Min(array=w26) -> (max value=w27:dbl)  [unwired: 3 out]
  n97 = call "NR_DeRateMatch.vi"("appended path"=w39, "deiwdata"=w104, "coded_data"=w100, "vnum"=w103, "prb_num"=w80, "error in (no error)"=w160, "rvid"=w102, "Qm"=w101, "EN_LDPC"=w95, "null_pos"=w99, "LDPC_base_graph"=w74, "Zc"=w96, "C"=w93, "Nsym_slot"=w90, "DMRS_symbol"=w97) -> ("dermdata"=w98:dbl[][], "error IO"=w159:errorcluster)  [unwired: 3 in]
  n98 = Round Toward +Infinity(x=w27) -> (ceil(x): smallest int >= x=w20:dbl)
  n99 = Multiply(x=w20, y=-1.0) -> (x*y=w21:dbl)
  n100 = call "NR_LDPC_Decode_opti.vi"("appended path"=w39, "Zc"=w96, "LDPC_base_graph"=w74, "C"=w93, "cdblkseg_data"=w75, "dermdata"=w98, "EN_LDPC"=w95, "error in (no error)"=w159) -> ("deldpccode"=w94:dbl[][], "error IO"=w146:errorcluster)  [unwired: 6 in]
  n101 = property on="接收端星座图" class="XYGraph (严格)"("XScale.Maximum"=w20, "XScale.Minimum"=w21, "YScale.Maximum"=w20, "YScale.Minimum"=w21) -> ()  [unwired: 2 in, 2 out]
  n102 = call "DeCRC.vi"("F"=w92, "error in (no error)"=w146, "deldpccode"=w94, "C"=w93, "appended path"=w39) -> ("error IO"=w84:errorcluster, "tbdata"=w1:dbl[], "crcflag"=w19:dbl)  [unwired: 4 in]
  n103 = Exclusive Or(1:w88, 2:w3) -> (0:w87:i32[])
  n104 = Array Size(array=w3) -> (size(s)=w4:i32)
  "总比特数（解调制映射输出数据）" <- w4
  n105 = Add Array Elements(numeric array=w87) -> (sum=w8:i32)
  "误码数（调制映射输入数据和解调制映射输出数据比较）" <- w8
  n106 = Exclusive Or(1:w85, 2:w1) -> (0:w86:i32[])
  n107 = Add Array Elements(numeric array=w86) -> (sum=w6:i32)
  "误码数（信源比特和信宿比特比较）" <- w6
  n108 = Build Path(base path=w39, name or relative path="rx_img.bmp" ("名称或相对路径")) -> (appended path=w40:path)
  n109 = call "NR_ReSourceData.vi"("imagrxpath"=w40, "error in (no error)"=w84, "tbdata"=w1, "appended path"=w39) -> ("imagrxpathout"=w68:path)  [unwired: 6 in, 1 out]
  n110 = case shown="1" w19 {
    tunnel: [FALSE ("CRC校验结果") TRUE ("CRC校验结果")] -> w18
    frame 0, Default {
    }
    frame 1 {
    }
  }
  "CRC校验结果" <- w18
  n111 = Divide(x=w8, y=w4) -> (x/y=→"误码率（调制映射输入数据和解调制映射输出数据比较）":dbl)
  n112 = call <vilib>:"Read BMP File.vi"("path to BMP file"=w68) -> ("image data"=w45:T7)  [unwired: 8 in, 2 out]
  n113 = Unbundle By Name(w45) -> ("Rectangle.right"=w48:i16, "Rectangle.bottom"=w47:i16)
  n114 = call <vilib>:"Draw Flattened Pixmap.vi"("image data"=w45) -> ("new picture"=→"接收图片":picture)  [unwired: 8 in]
  n115 = Bundle By Name(cluster=T4 {"Width"=0, "Height"=0} ("绘图区域大小"), "Width"=w48, "Height"=w47) -> (w44:T4)
  n116 = property on="接收图片" class="Pict"("Draw Area Size"=w44) -> ()  [unwired: 2 in, 2 out]
  n117 = Array Size(array=w1) -> (size(s)=w2:i32)
  "总比特数 （信宿比特）" <- w2
  n118 = Divide(x=w6, y=w2) -> (x/y=→"误码率（信源比特和信宿比特比较）":dbl)
